vi "Complex Add (SGL).vi"(8 "Input Valid":bool=TRUE, 10 "X2+j Y2":cluster{"Y2":fxp<+,32,32>, "X2":fxp<+,32,32>}, 11 "X1+j Y1":cluster{"Y1":fxp<+,32,32>, "X1":fxp<+,32,32>}) -> (0 "Output Valid":bool, 3 "Xout+j Yout":T1)   [LabVIEW 2011]
doc: "This VI performs single precision complex add\n\n<b> Latency = 11 Ticks </b>"
types:
  T1 = cluster{"Yout":fxp<+,32,32>, "Xout":fxp<+,32,32>}
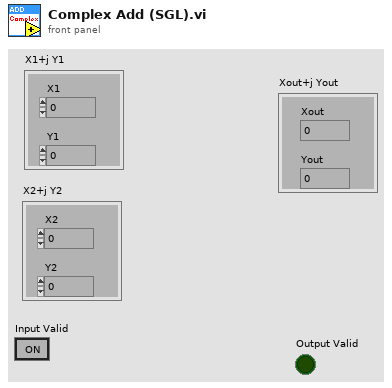
[diagram p1: front panel]
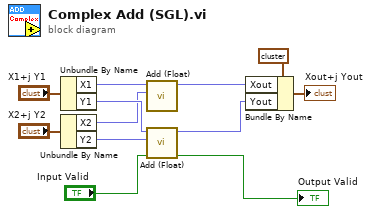
[diagram p0: block diagram]
diagram:
  n1 = Unbundle By Name("X1+j Y1") -> ("X1"=w4:fxp<+,32,32>, "Y1"=w5:fxp<+,32,32>)
  n2 = Unbundle By Name("X2+j Y2") -> ("X2"=w3:fxp<+,32,32>, "Y2"=w6:fxp<+,32,32>)
  n3 = call <userlib>:"Add (Float).vi"("b"=w3, "a"=w4) -> ("a+b"=w2:fxp<+,32,32>)  [unwired: 8 in, 1 out]
  n4 = call <userlib>:"Add (Float).vi"("Input Valid"="Input Valid", "b"=w6, "a"=w5) -> ("Output Valid"=→"Output Valid":bool, "a+b"=w8:fxp<+,32,32>)  [unwired: 7 in]
  n5 = Bundle By Name(cluster=T1 {"Yout"=0.0, "Xout"=0.0} ("Xout+j Yout"), "Xout"=w2, "Yout"=w8) -> (→"Xout+j Yout":T1)
